vi "Save Recall List File.vi"(8 "error in (no error)":errorcluster, 9 "List Number (1)":i32=1 min=1 max=7 format="%#_0f", 10 "Save Recall List File (0:Save)":u16(ring) items=["Save", "Recall"], 11 "VISA resource name":refnum<visa-resource-name>) -> (0 "error out":errorcluster, 3 "VISA resource name out":refnum<visa-resource-name>)   [LabVIEW 2018, in "BK Precision 8600 Series.lvlib"]
doc: "Saves or recalls a list file. A list file contains all programmed list step parameters and list operation parameters from <b>Configure List Operation.vi</b> and <b>Configure List Step Parameters.vi</b>.\n\nIf saving a list file, run this after all list step parameters are configured."
uses:
  <instrlib>/BK Precision 8600 Series/BK Precision 8600 Series.lvlib
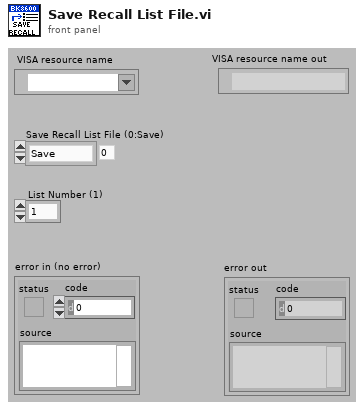
[diagram p1: front panel]
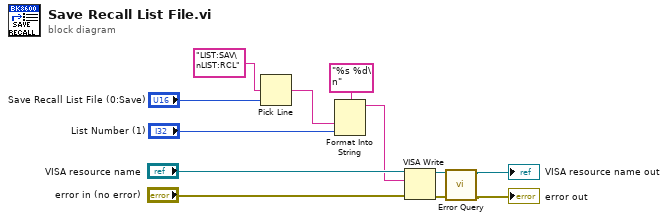
[diagram p0: block diagram]
diagram:
  n1 = Pick Line(multi-line string="LIST:SAV\nLIST:RCL", line index="Save Recall List File (0:Save)") -> (output string=w8:string)  [unwired: 1 in]
  n2 = Format Into String(format string="%s %d\n", w8, "List Number (1)") -> (resulting string=w5:string)  [unwired: 2 in, 1 out]
  n3 = VISA Write(VISA resource name="VISA resource name", write buffer=w5, error in (no error)="error in (no error)") -> (VISA resource name out=w4:refnum<visa-resource-name>, error out=w3:errorcluster)  [unwired: 1 out]
  n4 = call <instrlib>:"Error Query.vi"("error in (no error)"=w3, "VISA resource name"=w4) -> ("error out"=→"error out":errorcluster, "VISA resource name out"=→"VISA resource name out":refnum<visa-resource-name>)  [unwired: 6 in, 2 out]
